vi "Write Delimited.vi"() -> ()   [LabVIEW 2022 SP3]
uses:
  <vilib>/Utility/file.llb/Write Delimited Spreadsheet (string).vi
panel:
  in  "file path (dialog if empty)":path
  out "appended array 2":string[][](array[string])
  out "transposed array":string[][](array[string])
  out "appended array":string[][](array[string])
  in  "Array 3":string[](array[string])
  in  "Array 2":string[](array[string])
  out "F-format string":string[][](array[string])
  out "Array":dbl[][](array[numeric])
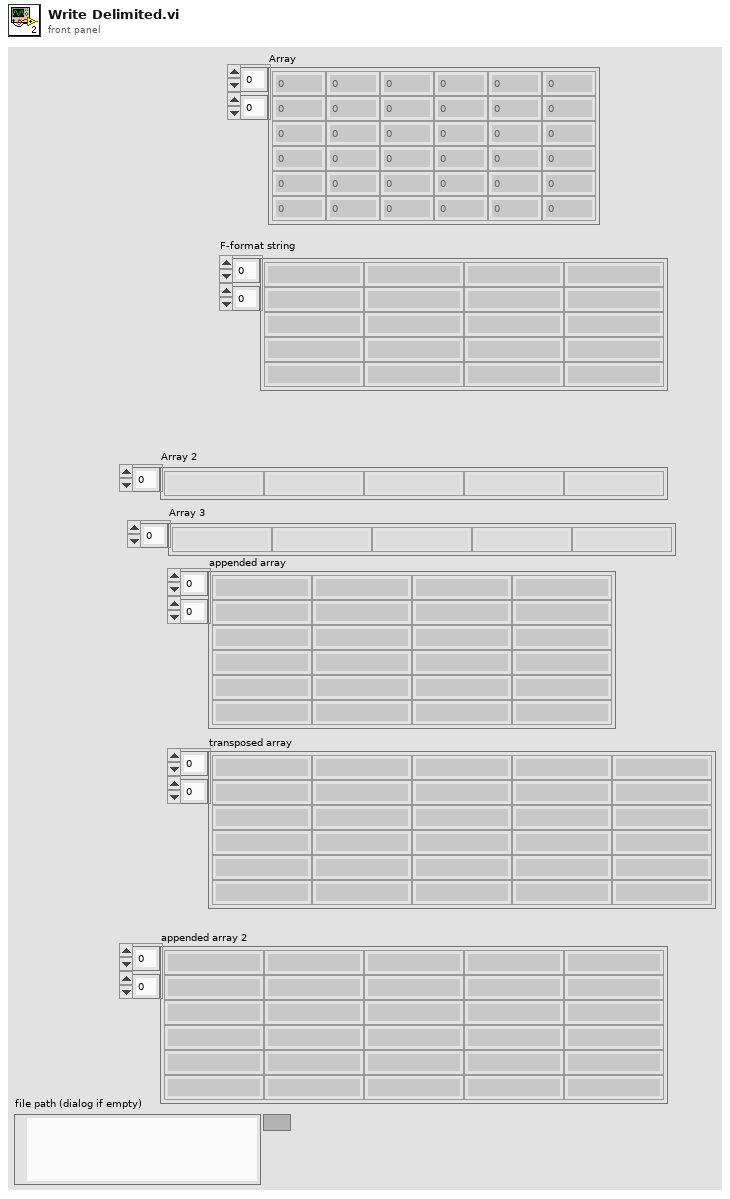
[diagram p1: front panel]
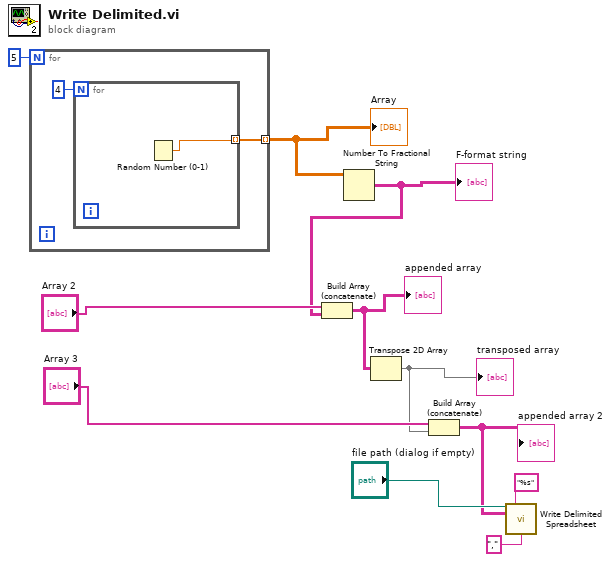
[diagram p0: block diagram]
diagram:
  n1 = for {
    N: 5 -> [_]
    tunnel: [w12] -> w10 mode=indexing
    n2 = for {
      N: 4 -> [_]
      tunnel: [w14] -> w12 mode=indexing
      n3 = Random Number (0-1)() -> (number: 0 to 1=w14:dbl)
    }
  }
  "Array" <- w10
  n4 = Number To Fractional String(number=w10) -> (F-format string=w8:string[][])  [unwired: 3 in]
  "F-format string" <- w8
  n5 = Build Array (concatenate)("Array 2", w8) -> (w7:string[][])
  "appended array" <- w7
  n6 = Transpose 2D Array(2D array=w7) -> (transposed array=w5:string[][])
  "transposed array" <- w5
  n7 = Build Array (concatenate)("Array 3", w5) -> (w3:string[][])
  "appended array 2" <- w3
  n8 = call-poly <vilib>:"Write Delimited Spreadsheet.vi"("file path (dialog if empty)"="file path (dialog if empty)", "format (%s)"="%s", "2D data"=w3, "delimiter (\\t)"="," ("delimiter (\\t)")) -> ()  [unwired: 10 in, 2 out]
